vi "fetch_and_translate_trigger.vi"(8 "error in (no error)":errorcluster, 11 "ScanHeadAK130114ResonanceFlexRIO in":refnum<class "ScanHeadAK130114ResonanceFlexRIO.lvclass">) -> (0 "error out":errorcluster, 1 "sender TLC type":T2, 2 "internal trigger":T1, 3 "ScanHeadAK130114ResonanceFlexRIO out":refnum<class "ScanHeadAK130114ResonanceFlexRIO.lvclass">)   [LabVIEW 2010, in "ScanHeadAK130114ResonanceFlexRIO.lvclass"]
uses:
  ScanHeadAK130114ResonanceFlexRIO.lvclass
  common/enumerations/top-level_component_type_enum.ctl
  internal_trigger_enum.ctl
  GenericScanHead/GenericScanHead/trigger_enum.ctl
  GenericScanHead/GenericScanHead/GenericScanHead.lvclass
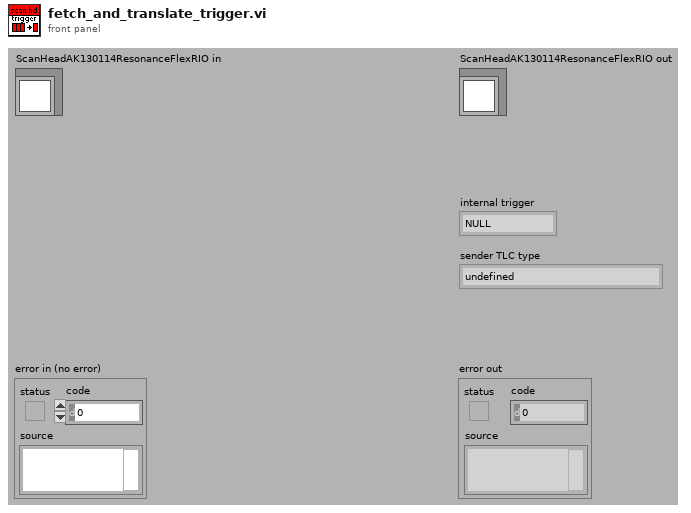
[diagram p1: front panel]
types:
  T1 = typedef "ScanHeadAK130114ResonanceFlexRIO.lvclass/internal_trigger_enum.ctl" = enum16{"NULL", "initialise", "terminate", "start scanning", "stop scanning", "update", "fetch trajectory"}
  T2 = typedef "top-level_component_type_enum.ctl" = enum16{"undefined", "ImagingMode", "ScanHead", "DAQ", "ImageAssembler", "Display", "DataCollection", "Analyser", "Stimulator", "ExperimentController", "Instrument", "Stage"}
  T3 = typedef "GenericScanHead.lvclass/trigger_enum.ctl" = enum16{"NULL", "fetch trajectory", "generate trajectory", "change run mode", "update modifiers"}
  T4 = typedef "GenericToplevelComponent.lvclass/common_trigger_enum.ctl" = enum16{"NULL", "initialise", "terminate", "fetch command", "fetch data", "attach observer", "register as observer", "detach observer", "acknowledge", "start", "stop", "sweep started", "sweep finished", "experiment started", "experiment stopped"}
  T5 = typedef "trigger_type_enum.ctl" = enum8{"external", "internal", "common"}
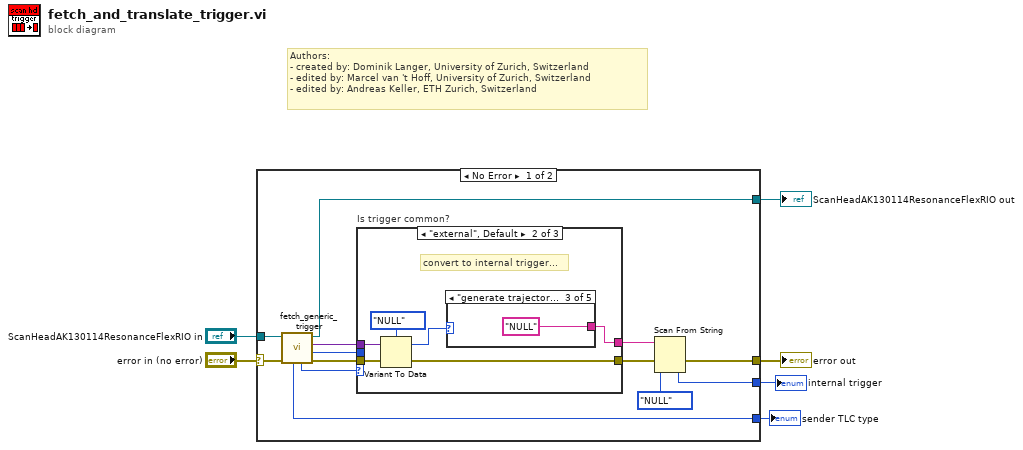
[diagram p0: block diagram]
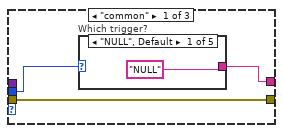
[diagram p2: hidden frame]
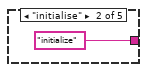
[diagram p3: hidden frame]
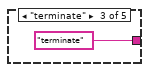
[diagram p4: hidden frame]
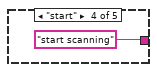
[diagram p5: hidden frame]
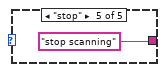
[diagram p6: hidden frame]
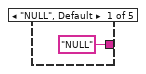
[diagram p7: hidden frame]
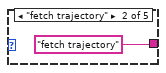
[diagram p8: hidden frame]
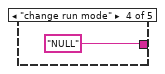
[diagram p9: hidden frame]
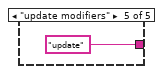
[diagram p10: hidden frame]
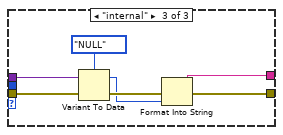
[diagram p11: hidden frame]
diagram:
  # "Authors: \n- created by: Dominik Langer, University of Zurich, Switzerland\n- edited by: Marcel van 't Hoff, University of Zurich, Switzerland\n- edited by: Andreas Keller, ETH Zurich, Switzerland"
  n1 = case shown="No Error" "error in (no error)" {
    selector: "error in (no error)" -> [w14 w47]
    tunnel: [w15 w47] -> w5
    tunnel: [w10 w46] -> w3
    tunnel: "ScanHeadAK130114ResonanceFlexRIO in" -> [w11 w46]
    tunnel: [w9 _] -> w1
    tunnel: [w8 _] -> w2
    frame No Error {
      n2 = call-dynamic "fetch_generic_trigger.vi"("error in (no error)"=w14, "GenericToplevelComponent in"=w11) -> ("error out"=w17:errorcluster, "common trigger"=w18:T4, "trigger"=w13:variant, "GenericToplevelComponent out"=w10:refnum<class "ScanHeadAK130114ResonanceFlexRIO.lvclass">, "trigger type"=w19:T5, "sender TLC type"=w8:T2)  [unwired: 3 in, 1 out]
      n3 = case "Is trigger common?" shown="\"external\", Default" w19 {
        tunnel: w18 -> [w22 _ _]
        tunnel: w17 -> [w21 w32 w43]
        tunnel: [w21 w30 w42] -> w16
        tunnel: w13 -> [_ w33 w45]
        tunnel: [w20 w29 w40] -> w12
        frame "common" {
          n4 = case "Which trigger?" shown="\"NULL\", Default" w22 {
            tunnel: ["NULL" "initialize" "terminate" "start scanning" "stop scanning"] -> w20
            frame "NULL", Default {
            }
            frame "initialise" {
            }
            frame "terminate" {
            }
            frame "start" {
            }
            frame "stop" {
            }
          }
        }
        frame "external", Default {
          # "convert to internal trigger..."
          n5 = Variant To Data(error in=w32, Variant=w33, type=trigger_enum."NULL" ("trigger")) -> (error out=w30:errorcluster, data=w31:T3)
          n6 = case shown="\"generate trajectory\"" w31 {
            tunnel: ["NULL" "fetch trajectory" "NULL" "NULL" "update"] -> w29
            frame "NULL", Default {
            }
            frame "fetch trajectory" {
            }
            frame "generate trajectory" {
            }
            frame "change run mode" {
            }
            frame "update modifiers" {
            }
          }
        }
        frame "internal" {
          n7 = Variant To Data(error in=w43, Variant=w45, type=internal_trigger_enum."NULL" ("trigger")) -> (error out=w44:errorcluster, data=w41:T1)
          n8 = Format Into String(error in=w44, w41) -> (resulting string=w40:string, error out=w42:errorcluster)  [unwired: 2 in]
        }
      }
      n9 = Scan From String(input string=w12, error in=w16, default 1=internal_trigger_enum."NULL" ("trigger")) -> (error out=w15:errorcluster, output 1=w9:T1)  [unwired: 2 in, 2 out]
    }
    frame Error {
    }
  }
  "error out" <- w5
  "ScanHeadAK130114ResonanceFlexRIO out" <- w3
  "sender TLC type" <- w2
  "internal trigger" <- w1
